vi "Compact Color Map.vi"(7 "X Dimension":i32, 10 "Color Index Array In":i32[](array[numeric]), 11 "Vertex Array In":cluster{"X":sgl, "Y":sgl, "Z":sgl}[](array[cluster])) -> (1 "Index for Same Color Vertex":u32[](array[numeric]), 2 "Compact Color Index Array Out":i32[](array[numeric]), 3 "Reordered Vertex Array Out":cluster{"X":sgl, "Y":sgl, "Z":sgl}[](array[cluster]))   [LabVIEW 2020, in "3D Plot Datatype.lvclass"]
uses:
  <vilib>/Math Plots/3D Math Plots/3D Plot/3D Plot Datatype/3D Plot Datatype.lvclass
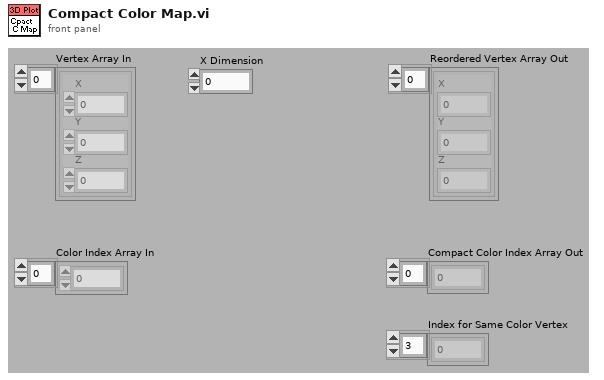
[diagram p1: front panel]
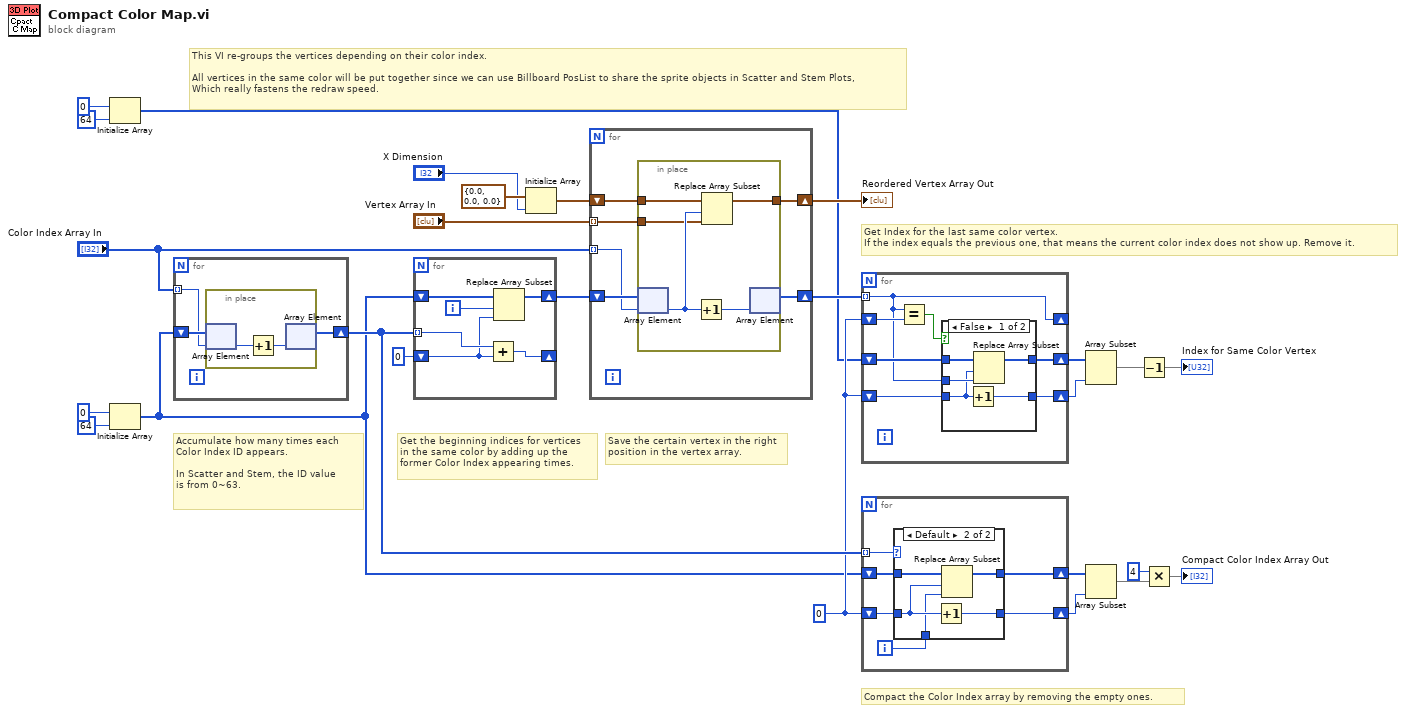
[diagram p0: block diagram]
diagram:
  w5 = 0
  # "Compact the Color Index array by removing the empty ones."
  # "Get Index for the last same color vertex.\nIf the index equals the previous one, that means the current color index does not show up. Remove it."
  # "Save the certain vertex in the right\nposition in the vertex array."
  # "This VI re-groups the vertices depending on their color index. \n\nAll vertices in the same color will be put together since we can use Billboard PosList to share the sprite objects in Scatter and Stem Plots,\nWhich really fastens the redraw speed."
  # "Get the beginning indices for vertices\nin the same color by adding up the \nformer Color Index appearing times."
  # "Accumulate how many times each \nColor Index ID appears.\n\nIn Scatter and Stem, the ID value \nis from 0~63."
  n1 = Initialize Array(u32 0, 64 ("dimension size")) -> (w1:u32[])
  n2 = Initialize Array(0, 64 ("dimension size")) -> (w4:i32[])
  n3 = for {
    tunnel: "Color Index Array In" -> [w28] mode=indexing
    shift-right: [w27] -> w6
    shift-left: w4 -> [w29]
    n4 = in-place {
      n5 = in-place-array #1(w29, w28) -> (w31:i32)
      n6 = Increment(x=w31) -> (x+1=w30:i32)
      n7 = in-place-array #1(w30) -> (w27:i32[])  [unwired: 1 out]
    }
  }
  n8 = for {
    shift-right: [w34] -> w19
    shift-left: w4 -> [w35]
    shift-right: [w37] -> _
    shift-left: 0 -> [w32]
    tunnel: w6 -> [w36] mode=indexing
    i -> [w33]
    n9 = Add(x=w36, y=w32) -> (x+y=w37:i32)
    n10 = Replace Array Subset(array=w35, new element=w32, index=w33) -> (w34:i32[])
  }
  n11 = Initialize Array(cluster{"X":sgl, "Y":sgl, "Z":sgl} {"X"=0.0, "Y"=0.0, "Z"=0.0} ("3D Point 2"), "X Dimension") -> (w21:cluster{"X":sgl, "Y":sgl, "Z":sgl}[])
  n12 = for {
    tunnel: "Vertex Array In" -> [w42] mode=indexing
    shift-right: [w41] -> w9
    shift-left: w21 -> [w43]
    tunnel: "Color Index Array In" -> [w39] mode=indexing
    shift-right: [w38] -> w16
    shift-left: w19 -> [w40]
    n13 = in-place {
      in-place-border: w43 -> [w47]
      in-place-border: w42 -> [w44]
      in-place-border: [w46] -> w41
      n14 = in-place-array #2(w40, w39) -> (w45:i32)
      n15 = Increment(x=w45) -> (x+1=w48:i32)
      n16 = Replace Array Subset(array=w47, new element=w44, index=w45) -> (w46:cluster{"X":sgl, "Y":sgl, "Z":sgl}[])
      n17 = in-place-array #2(w48) -> (w38:i32[])  [unwired: 1 out]
    }
  }
  "Reordered Vertex Array Out" <- w9
  n18 = for {
    tunnel: w16 -> [w51] mode=indexing
    shift-right: [w52] -> w15
    shift-left: w1 -> [w53]
    shift-right: [w51] -> _
    shift-left: w5 -> [w55]
    shift-right: [w49] -> w14
    shift-left: w5 -> [w50]
    n19 = Equal?(x=w51, y=w55) -> (x = y?=w54:bool)
    n20 = case shown="False" w54 {
      tunnel: w53 -> [w60 w62]
      tunnel: [w59 w62] -> w52
      tunnel: w51 -> [w58 _]
      tunnel: w50 -> [w56 w61]
      tunnel: [w57 w61] -> w49
      frame False {
        n21 = Increment(x=w56) -> (x+1=w57:i32)
        n22 = Replace Array Subset(array=w60, new element=w58, index=w56) -> (w59:u32[])
      }
      frame True {
      }
    }
  }
  n23 = for {
    tunnel: w6 -> [w68] mode=indexing
    shift-right: [w66] -> w18
    shift-left: w4 -> [w67]
    shift-right: [w65] -> w17
    shift-left: w5 -> [w64]
    i -> [w63]
    n24 = case shown="Default" w68 {
      tunnel: w67 -> [w70 w75]
      tunnel: [w70 w74] -> w66
      tunnel: [w69 w73] -> w65
      tunnel: w64 -> [w69 w72]
      tunnel: w63 -> [_ w71]
      frame 0 {
      }
      frame Default {
        n25 = Increment(x=w72) -> (x+1=w73:i32)
        n26 = Replace Array Subset(array=w75, new element=w71, index=w72) -> (w74:i32[])
      }
    }
  }
  n27 = Array Subset(array=w15, length=w14) -> (w13:u32[])  [unwired: 1 in]
  n28 = Array Subset(array=w18, length=w17) -> (w26:i32[])  [unwired: 1 in]
  n29 = Decrement(x=w13) -> (x-1=→"Index for Same Color Vertex":u32[])
  n30 = Multiply(x=4, y=w26) -> (x*y=→"Compact Color Index Array Out":i32[])
